vi "IZRCSMsettings_ut_test.vi"(8 "Error In":errorcluster, 11 "CSMinfo in":T1) -> (0 "Error Out":errorcluster, 3 "CSMinfo out":T1)   [LabVIEW 2018]
uses:
  IZRCSM.ctl
  MOKO_LabViewLibrary/MokoSTM/MokoClassicUtilitySTM/MCUS_STM.ctl
  MOKO_LabViewLibrary/MokoSTM/MokoClassicUtilitySTM/MCUS_ITEM.ctl
panel:
  in  "Verifier":string
  in  "Request":string
  in  "Owner":string
  in  "SerialNumber":string
  in  "ModelDevice":string
  in  "CurrentDate":string
  in  "ProtocolNumber":string
  in  "Применить":bool
  # "Registration"
  # "Protocol №:"
  # "Current date:"
  # "0,4\n0,6\n1\n1,5\n1,6\n2,5\n4"
  # "kPa\nbar\nkgf/cm2\nMPa"
  # "Model device:"
  # "Serial Numer:"
  # "Owner:"
  # "Request:"
  # "Verifier:"
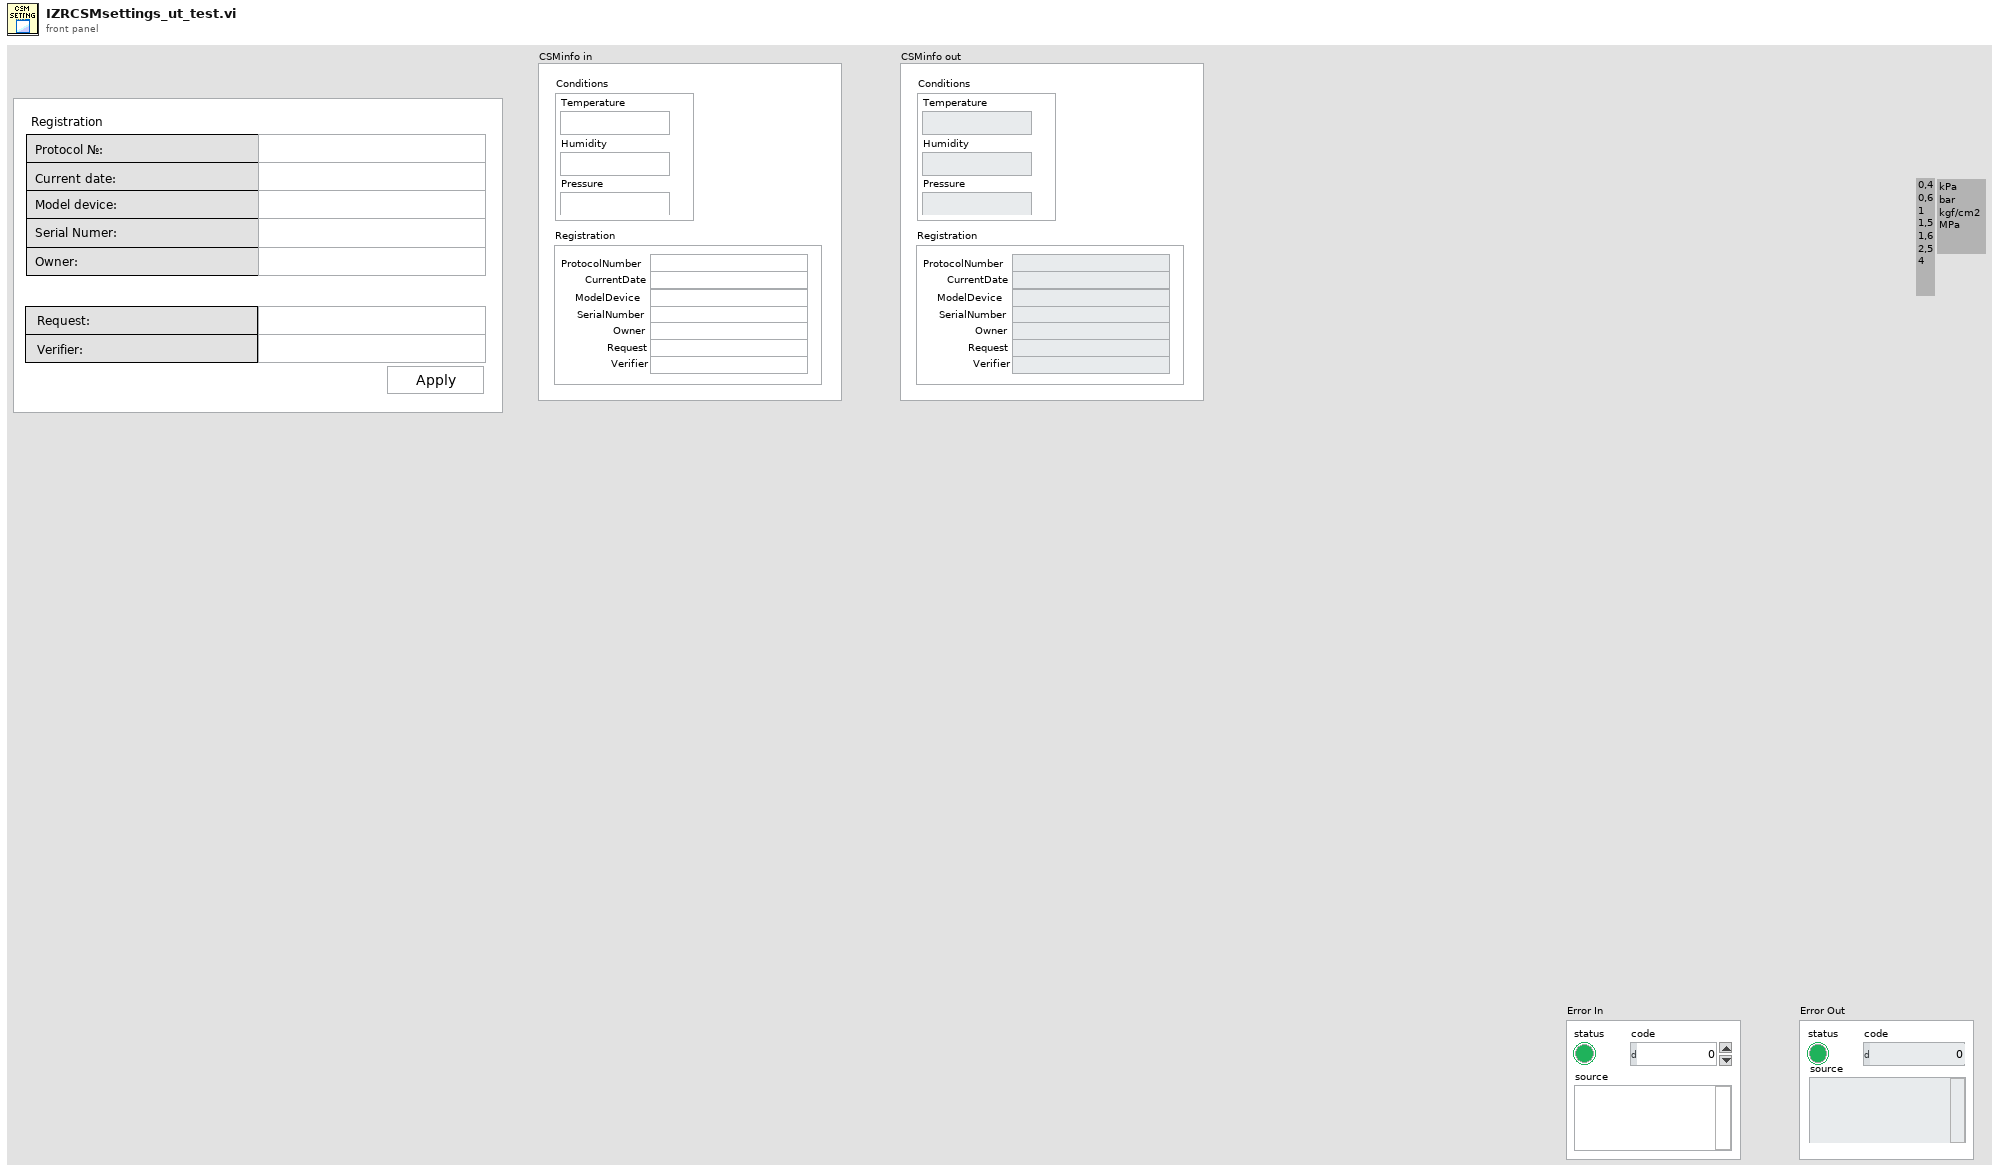
[diagram p1: front panel]
types:
  T1 = typedef "IZRCSM.ctl" = cluster{"Conditions":cluster{"Temperature":string, "Humidity":string, "Pressure":string}, "Registration":cluster{"ProtocolNumber":string, "CurrentDate":string, "ModelDevice":string, "SerialNumber":string, "Owner":string, "Request":string, "Verifier":string}}
  T2 = typedef "MCUS_STM.ctl" = cluster{"main stm":T3, "data":string}
  T3 = typedef "MCUS_ITEM.ctl" = enum16{"idle", "_____ main_____ ", "Init", "Stop", "Apply values", "Save", "Open", "Reset"}
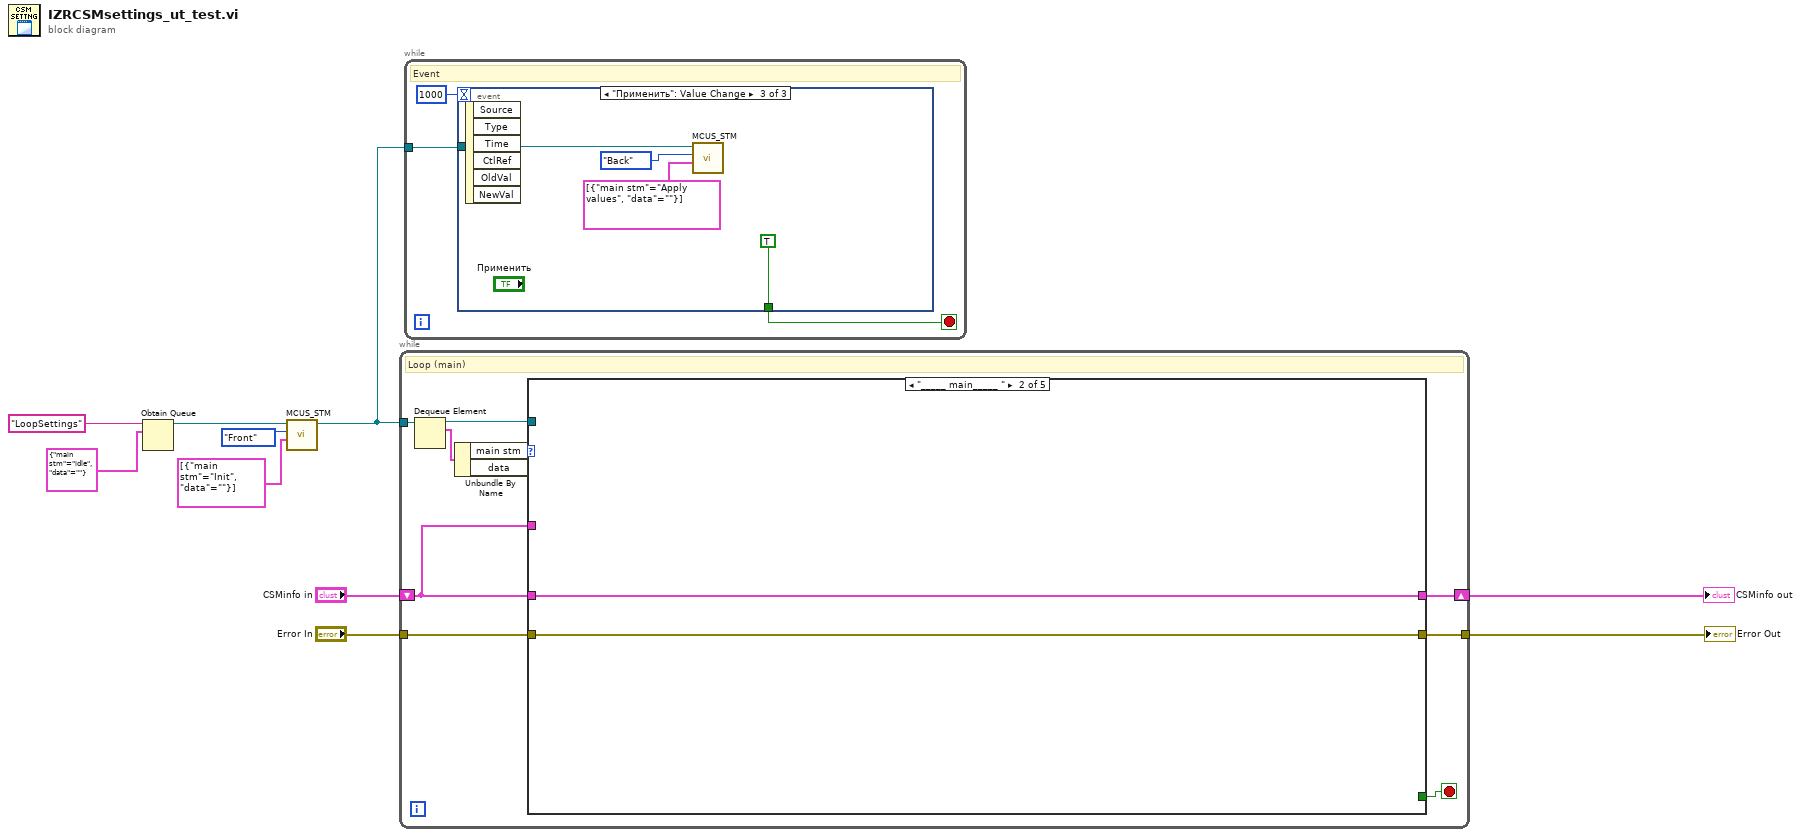
[diagram p0: block diagram]
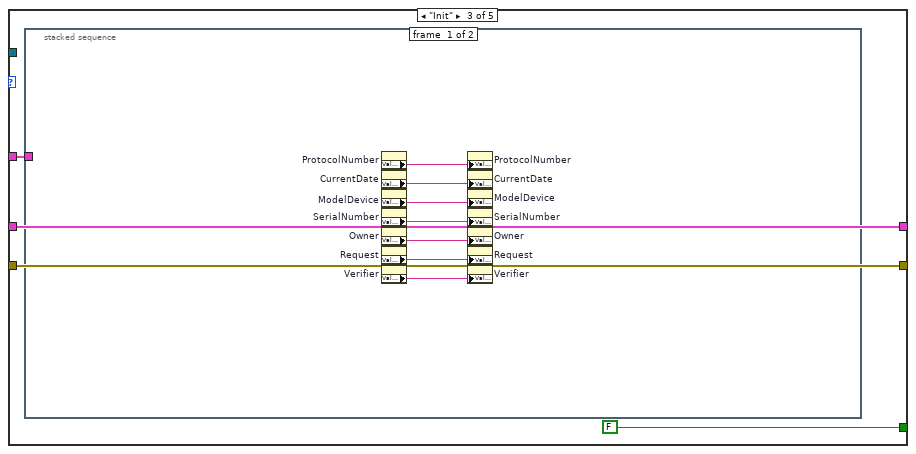
[diagram p3: hidden frame]
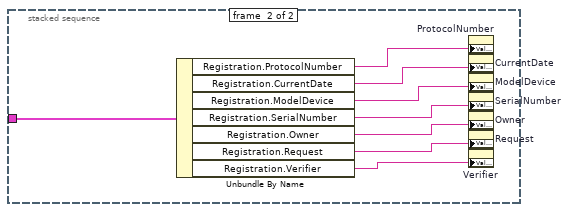
[diagram p4: hidden frame]
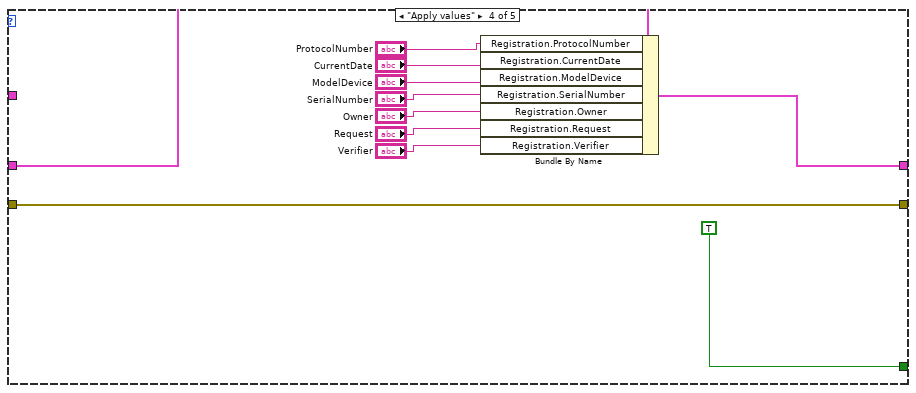
[diagram p5: hidden frame]
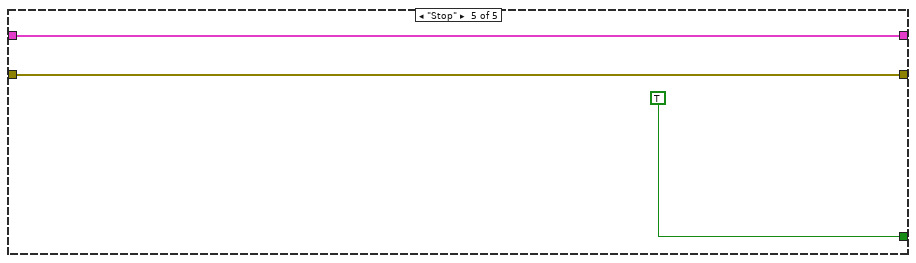
[diagram p6: hidden frame]
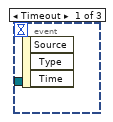
[diagram p7: hidden frame]
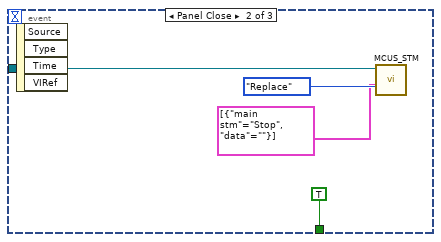
[diagram p8: hidden frame]
diagram:
  n1 = Obtain Queue(name (unnamed)="LoopSettings", element data type=T2 {"main stm"=enum."idle", "data"=""} ("MOKO_NMEA")) -> (queue out=w10:refnum<queue>)  [unwired: 3 in, 2 out]
  n2 = call "MCUS_STM.vi"("StateMachineSteps"=T2[] [{"main stm"=enum."Init", "data"=""}], "FNs"=enum16{"Back", "Front", "Replace"}."Front", "Queue in"=w10) -> ("Queue out"=w5:refnum<queue>)  [unwired: 7 in, 1 out]
  n3 = while {
    tunnel: w5 -> [w19]
    tunnel: "Error In" -> [w14]
    tunnel: [w13] -> w3
    shift-right: [w12] -> w1
    shift-left: "CSMinfo in" -> [w11]
    stop <- w15 stop-if-true
    # "Loop (main)"
    n4 = Dequeue Element(queue=w19) -> (queue out=w18:refnum<queue>, element=w17:T2)  [unwired: 2 in, 2 out]
    n5 = Unbundle By Name(w17) -> ("main stm"=w16:T3)  [unwired: 1 out]
    n6 = case shown="\"_____ main_____ \"" w16 {
      tunnel: w18 -> [_ _ _ _ _]
      tunnel: [_ _ FALSE TRUE TRUE] -> w15
      tunnel: w14 -> [w20 w22 w27 w53 w56]
      tunnel: [w20 w22 w27 w53 w56] -> w13
      tunnel: [w21 w23 w25 w50 w55] -> w12
      tunnel: w11 -> [w21 w23 w25 w51 w55]
      tunnel: w11 -> [_ _ w24 _ _]
      frame "idle", Default {
      }
      frame "_____ main_____ " {
      }
      frame "Init" {
        n7 = stacked-sequence {
          tunnel: w24 -> [_ w42]
          frame #0 {
            n8 = property on="ProtocolNumber" class="Str"() -> ("Value"=w34:string)  [unwired: 2 in, 2 out]
            n9 = property on="CurrentDate" class="Str"() -> ("Value"=w33:string)  [unwired: 2 in, 2 out]
            n10 = property on="ModelDevice" class="Str"() -> ("Value"=w32:string)  [unwired: 2 in, 2 out]
            n11 = property on="SerialNumber" class="Str"() -> ("Value"=w31:string)  [unwired: 2 in, 2 out]
            n12 = property on="Owner" class="Str"() -> ("Value"=w30:string)  [unwired: 2 in, 2 out]
            n13 = property on="Request" class="Str"() -> ("Value"=w29:string)  [unwired: 2 in, 2 out]
            n14 = property on="Verifier" class="Str"() -> ("Value"=w28:string)  [unwired: 2 in, 2 out]
            n15 = property on="ProtocolNumber" class="Str"("Value"=w34) -> ()  [unwired: 2 in, 2 out]
            n16 = property on="CurrentDate" class="Str"("Value"=w33) -> ()  [unwired: 2 in, 2 out]
            n17 = property on="ModelDevice" class="Str"("Value"=w32) -> ()  [unwired: 2 in, 2 out]
            n18 = property on="SerialNumber" class="Str"("Value"=w31) -> ()  [unwired: 2 in, 2 out]
            n19 = property on="Owner" class="Str"("Value"=w30) -> ()  [unwired: 2 in, 2 out]
            n20 = property on="Request" class="Str"("Value"=w29) -> ()  [unwired: 2 in, 2 out]
            n21 = property on="Verifier" class="Str"("Value"=w28) -> ()  [unwired: 2 in, 2 out]
          }
          frame #1 {
            n22 = Unbundle By Name(w42) -> ("Registration.ProtocolNumber"=w41:string, "Registration.CurrentDate"=w40:string, "Registration.ModelDevice"=w39:string, "Registration.SerialNumber"=w38:string, "Registration.Owner"=w37:string, "Registration.Request"=w36:string, "Registration.Verifier"=w35:string)
            n23 = property on="ProtocolNumber" class="Str"("Value"=w41) -> ()  [unwired: 2 in, 2 out]
            n24 = property on="CurrentDate" class="Str"("Value"=w40) -> ()  [unwired: 2 in, 2 out]
            n25 = property on="ModelDevice" class="Str"("Value"=w39) -> ()  [unwired: 2 in, 2 out]
            n26 = property on="SerialNumber" class="Str"("Value"=w38) -> ()  [unwired: 2 in, 2 out]
            n27 = property on="Owner" class="Str"("Value"=w37) -> ()  [unwired: 2 in, 2 out]
            n28 = property on="Request" class="Str"("Value"=w36) -> ()  [unwired: 2 in, 2 out]
            n29 = property on="Verifier" class="Str"("Value"=w35) -> ()  [unwired: 2 in, 2 out]
          }
        }
      }
      frame "Apply values" {
        n30 = Bundle By Name(cluster=w51, "Registration.ProtocolNumber"="ProtocolNumber", "Registration.CurrentDate"="CurrentDate", "Registration.ModelDevice"="ModelDevice", "Registration.SerialNumber"="SerialNumber", "Registration.Owner"="Owner", "Registration.Request"="Request", "Registration.Verifier"="Verifier") -> (w50:T1)
      }
      frame "Stop" {
      }
    }
  }
  "CSMinfo out" <- w1
  "Error Out" <- w3
  n31 = while {
    tunnel: w5 -> [w57]
    stop <- w59 stop-if-true
    # "Event"
    n32 = event shown="[2] \"Применить\": Value Change" {
      selector: _ -> [_ _ _]
      dyn-events: _ -> [_ _ _]
      timeout: 1000 -> [_ _ _]
      tunnel: [_ TRUE TRUE] -> w59
      tunnel: w57 -> [_ w60 w65]
      event Timeout {
        n33 = event-data() -> ()  [unwired: 1 in, 3 out]
      }
      event Panel Close {
        n34 = event-data() -> ()  [unwired: 1 in, 4 out]
        n35 = call "MCUS_STM.vi"("StateMachineSteps"=T2[] [{"main stm"=enum."Stop", "data"=""}], "FNs"=enum16{"Back", "Front", "Replace"}."Replace", "Queue in"=w60) -> ()  [unwired: 7 in, 2 out]
      }
      event "Применить": Value Change {
        n36 = event-data() -> ()  [unwired: 1 in, 6 out]
        n37 = call "MCUS_STM.vi"("StateMachineSteps"=T2[] [{"main stm"=enum."Apply values", "data"=""}], "FNs"=enum16{"Back", "Front", "Replace"}."Back", "Queue in"=w65) -> ()  [unwired: 7 in, 2 out]
      }
    }
  }
